vi "Indicacion.vi"(1 "Pos Elevator":i32) -> (0 "Indicacion":i32)   [LabVIEW 2018]
doc: "Este vi se encarga de la indicacion een el display del ascensor"
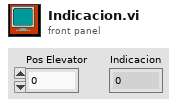
[diagram p1: front panel]
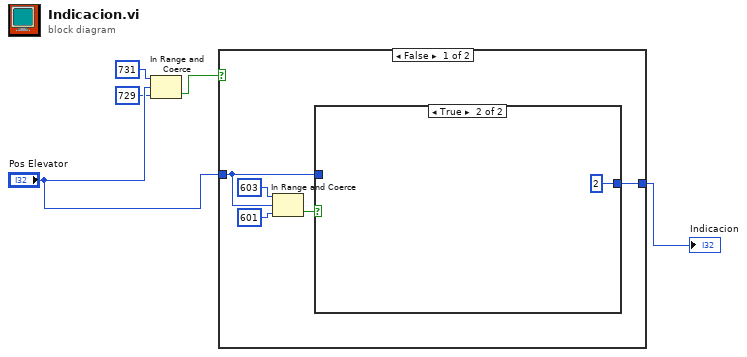
[diagram p0: block diagram]
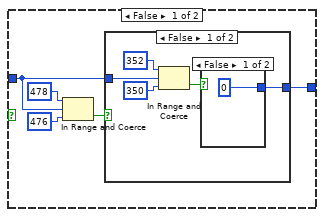
[diagram p2: hidden frame]
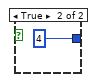
[diagram p3: hidden frame]
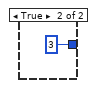
[diagram p4: hidden frame]
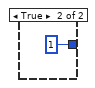
[diagram p5: hidden frame]
diagram:
  n1 = In Range and Coerce(upper limit=731, x="Pos Elevator", lower limit=729 ("upper limit")) -> (In Range?=w3:bool)  [unwired: 1 out]
  n2 = case shown="False" w3 {
    tunnel: [w6 1 ("upper limit")] -> w4
    tunnel: "Pos Elevator" -> [w7 _]
    frame False {
      n3 = In Range and Coerce(upper limit=603, x=w7, lower limit=601 ("upper limit")) -> (In Range?=w8:bool)  [unwired: 1 out]
      n4 = case shown="True" w8 {
        tunnel: [w12 2 ("upper limit")] -> w6
        tunnel: w7 -> [w11 _]
        frame False {
          n5 = In Range and Coerce(upper limit=478, x=w11, lower limit=476 ("upper limit")) -> (In Range?=w13:bool)  [unwired: 1 out]
          n6 = case shown="False" w13 {
            tunnel: [w16 3 ("upper limit")] -> w12
            tunnel: w11 -> [w18 _]
            frame False {
              n7 = In Range and Coerce(upper limit=352, x=w18, lower limit=350 ("upper limit")) -> (In Range?=w17:bool)  [unwired: 1 out]
              n8 = case shown="False" w17 {
                tunnel: [0 ("upper limit") 4 ("upper limit")] -> w16
                frame False {
                }
                frame True {
                }
              }
            }
            frame True {
            }
          }
        }
        frame True {
        }
      }
    }
    frame True {
    }
  }
  "Indicacion" <- w4
